vi "EKG.vi"() -> ()   [LabVIEW 2022 SP3]
uses:
  ViewData/-ReadEye/TypeDefs/TypeofMean.ctl
  <vilib>/Analysis/3filter.llb/Filter Passband Type.ctl
  <vilib>/Analysis/3filter.llb/Savitzky-Golay Filter (DBL).vi
  <vilib>/Analysis/baseanly.llb/Scale 1D.vi
  <vilib>/Utility/file.llb/Read Delimited Spreadsheet (string).vi
  <vilib>/picture/picture.llb/Draw True-Color Pixmap.vi
  <vilib>/Utility/file.llb/Write Delimited Spreadsheet (string).vi
  <vilib>/Analysis/NI_AAL_SigProc.lvlib
  <vilib>/Analysis/NI_AALBase.lvlib
panel:
  out "BPM file":string[][](array[string])
  out "clean lead 2 long":dbl[](graph)
  out "number of cycles":i32
  in  "Save?":bool
  out "clean lead 3":dbl[](graph)
  out "appended array":string[][](array[string])
  in  "Plot length":i32=3000
  in  "plot start":i32
  out "Input":dbl[](graph)
  out "Cycles":i32[](array[numeric])
  out "beats":i32
  in  "width":i32=10 min=3
  in  "Slide":dbl(slide)=0.5353535353535354 scale=0.0..1.0
  in  "slope correct?":bool
  in  "Process Path":path=path "\\\\vantage-n-wk\\H/Indus physiology recordings Fhf2 mouse"
  out "BPM":dbl
  in  "heartbeats":dbl=3.0
  out "Save Lead2":cluster{dbl[], "Y=(X-offset)/scale":dbl[]}(graph)
  out "clean Lead 3":cluster{dbl[], "Y=(X-offset)/scale":dbl[]}(graph)
  out "clean Lead 2":cluster{dbl[], "Y=(X-offset)/scale":dbl[]}(graph)
  out "Lead1":cluster{dbl[], "Y=(X-offset)/scale":dbl[]}(graph)
  in  "length":i32=6000
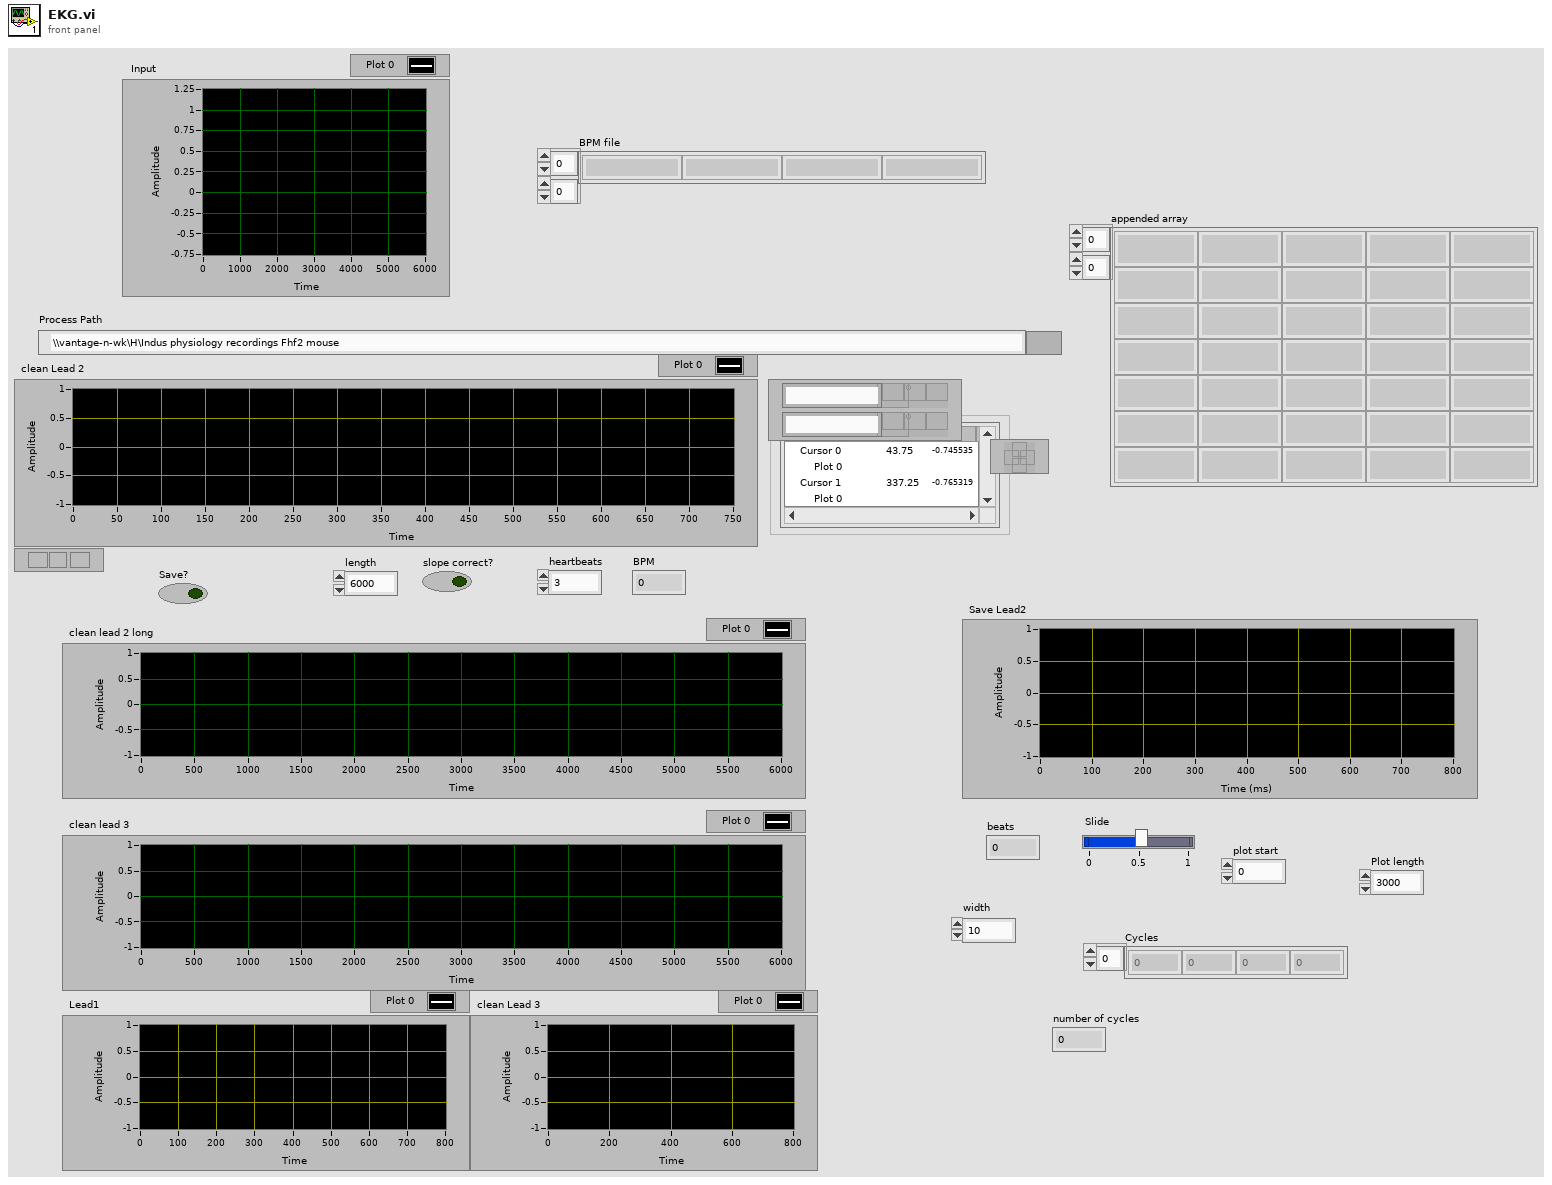
[diagram p1: front panel]
types:
  T1 = typedef "TypeofMean.ctl" = enum16{"Mean from lines", "Mean just lines", "Poly Mean", "No mean", "Filter"}
  T2 = typedef "NI_AALBase.lvlib/Filter Passband Type.ctl" = enum32{"Lowpass", "Highpass", "Bandpass", "Bandstop"}
  T3 = typedef "imagedata.ctl" = cluster{"image type":i32, "image depth":i32, "image":u8[], "mask":u8[], "colors":u32[], "Rectangle":cluster{"left":i16, "top":i16, "right":i16, "bottom":i16}}
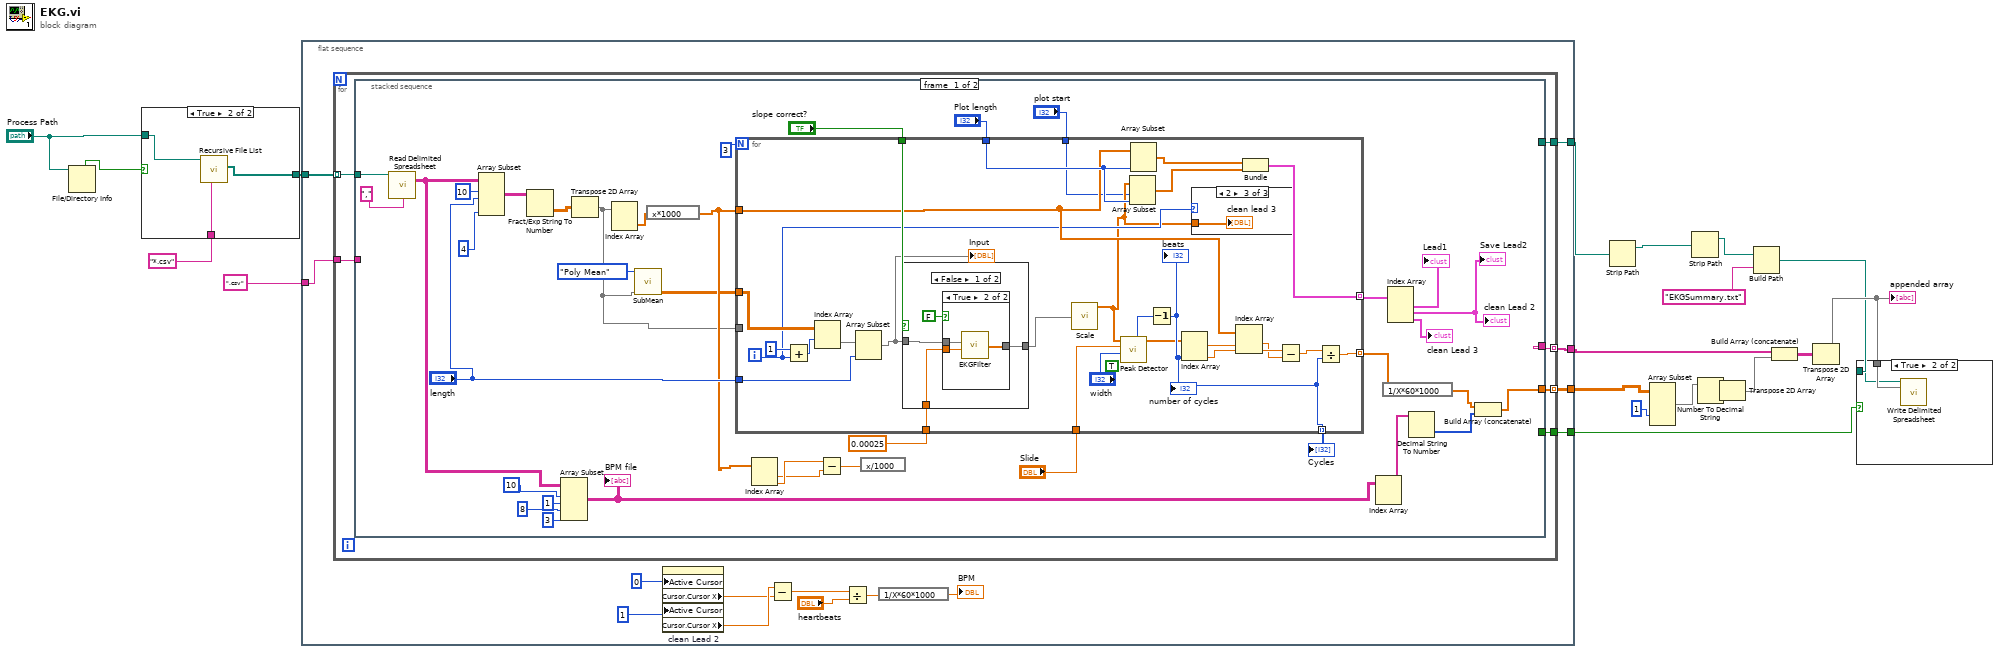
[diagram p0: block diagram]
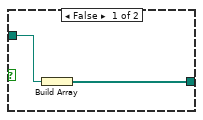
[diagram p3: hidden frame]
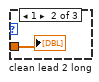
[diagram p5: hidden frame]
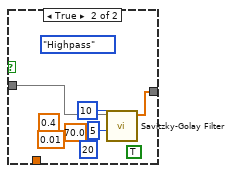
[diagram p7: hidden frame]
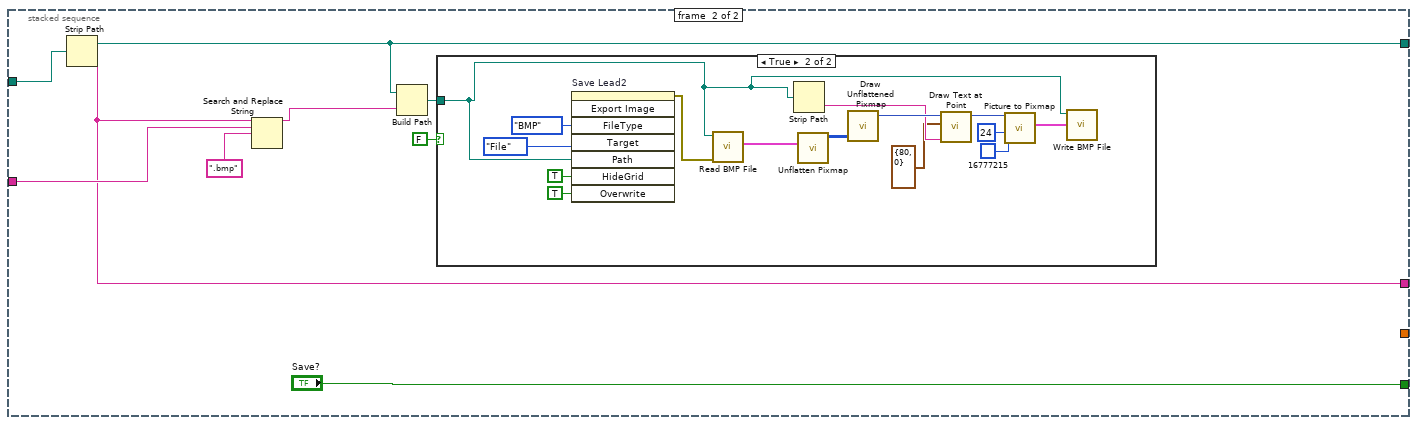
[diagram p8: hidden frame]
diagram:
  n1 = File/Directory Info(path="Process Path") -> (directory=w17:bool)  [unwired: 1 in, 6 out]
  n2 = case shown="True" w17 {
    tunnel: [w21 w24] -> w19
    tunnel: "Process Path" -> [w20 w23]
    tunnel: "*.csv" ("pattern") -> [_ w22]
    frame False {
      n3 = Build Array(w20) -> (w21:path[])
    }
    frame True {
      n4 = call <vilib>:"Recursive File List.vi"("pattern"=w22, "Folder Path"=w23) -> ("All Files in Dir"=w24:path[])  [unwired: 5 in, 4 out]
    }
  }
  n5 = flat-sequence {
    tunnel: w19 -> [w30]
    tunnel: [w26] -> w15
    tunnel: [w29] -> w14
    tunnel: [w28] -> w6
    tunnel: [w27] -> w2
    tunnel: ".csv" ("pattern") -> [w25]
    frame #0 {
      n6 = for {
        tunnel: w30 -> [w44] mode=indexing
        tunnel: [w43] -> w26 mode=indexing
        tunnel: w25 -> [w42]
        tunnel: [w41] -> w29 mode=indexing
        tunnel: [w40] -> w28
        tunnel: [w39] -> w27
        n7 = stacked-sequence {
          tunnel: w44 -> [w72 w132]
          tunnel: [w52 _] -> w43
          tunnel: w42 -> [_ w131]
          tunnel: [_ w127] -> w41
          tunnel: [_ w126] -> w40
          tunnel: [_ "Save?"] -> w39
          frame #0 {
            n8 = call-poly <vilib>:"Read Delimited Spreadsheet.vi"("file path (dialog if empty)"=w72, "delimiter (\\t)"="," ("delimiter (\\t)")) -> ("all rows"=w69:string[][])  [unwired: 8 in, 5 out]
            n9 = Array Subset(array=w69, index (row)=10 ("index"), length (row)="length", length (col)=4 ("length")) -> (w78:string[][])  [unwired: 1 in]
            n10 = Fract/Exp String To Number(string=w78) -> (number=w71:dbl[][])  [unwired: 3 in, 1 out]
            n11 = Array Subset(array=w69, index (row)=10, length (row)=1 ("length"), index (col)=8 ("disabled index (col)"), length (col)=3 ("length")) -> (w48:string[][])
            "BPM file" <- w48
            n12 = Transpose 2D Array(2D array=w71) -> (transposed array=w57:dbl[][])
            n13 = Index Array(array=w57) -> (element=w59:dbl[])  [unwired: 2 in]
            n14 = call "SubMean.vi"("Scan Data In"=w57, "Type of Mean"=TypeofMean."Poly Mean") -> ("Array"=w55:dbl[][])  [unwired: 4 in, 2 out]
            n15 = expression code="x*1000"(w59) -> (w58:dbl[])
            n16 = for {
              N: 3 -> [_]
              tunnel: w57 -> [_]
              tunnel: w58 -> [w88]
              tunnel: [w107] -> w76 mode=indexing
              tunnel: "length" -> [w105]
              tunnel: "slope correct?" -> [w104]
              tunnel: "Slide" -> [w103]
              tunnel: [w99] -> w66 mode=indexing
              tunnel: [w94] -> w65 mode=indexing
              tunnel: "plot start" -> [w83]
              tunnel: "Plot length" -> [w93]
              tunnel: 0.00025 -> [w82]
              tunnel: w55 -> [w86]
              i -> [w85]
              (unwired) TRUE ("initialize? (F)")
              n17 = Add(x=1, y=w85) -> (x+y=w108:i32)
              n18 = Index Array(array=w86, index (row)=w108) -> (element=w106:dbl[])  [unwired: 1 in]
              n19 = Array Subset(array=w106, length=w105) -> (w89:dbl[])  [unwired: 1 in]
              "Input" <- w89
              n20 = case shown="False" w104 {
                tunnel: [w114 w123] -> w87
                tunnel: w89 -> [w115 w122]
                tunnel: w82 -> [w113 _]
                frame False {
                  n21 = case shown="True" FALSE {
                    tunnel: w115 -> [w116 w119]
                    tunnel: [w116 w118] -> w114
                    tunnel: w113 -> [_ w117]
                    frame False {
                    }
                    frame True {
                      n22 = call "EKGFIlter.vi"("dt"=w117, "Input EKG"=w119) -> ("EKG Out"=w118:dbl[])  [unwired: 9 in]
                    }
                  }
                }
                frame True {
                  (unwired) 70.0 ("ripple(dB)")
                  (unwired) 20 ("order")
                  (unwired) 0.4 ("sampling freq: fs")
                  (unwired) TRUE ("init/cont (init:F)")
                  (unwired) 0.01 ("high cutoff freq: fh")
                  (unwired) Filter_Passband_Type."Highpass" ("filter type")
                  n23 = call-poly <vilib>:"Savitzky-Golay Filter.vi"("polynomial order"=5, "side points"=10, "X"=w122) -> ("Filtered X"=w123:dbl[])  [unwired: 7 in, 1 out]
                }
              }
              n24 = call-poly <vilib>:"Scale.vi"("X"=w87) -> ("Y=(X-offset)/scale"=w84:dbl[])  [unwired: 3 out]
              n25 = call <vilib>:"Peak Detector.vi"("width"="width", "threshold"=w103, "X"=w84) -> ("Locations"=w90:dbl[], "# found"=w101:i32)  [unwired: 4 in, 3 out]
              n26 = Array Subset(array=w84, index=w83, length=w93) -> (w91:dbl[])
              n27 = Array Subset(array=w88, length=w93) -> (w92:dbl[])  [unwired: 1 in]
              n28 = Decrement(x=w101) -> (x-1=w94:i32)
              "beats" <- w94
              n29 = Index Array(array=w90, index #2=w94) -> (element #1=w97:dbl, element #2=w98:dbl)  [unwired: 1 in]
              n30 = case shown="2" w85 {
                tunnel: w84 -> [_ w110 w111]
                frame 0, Default {
                }
                frame 1 {
                  "clean lead 2 long" <- w110
                }
                frame 2 {
                  "clean lead 3" <- w111
                }
              }
              n31 = Index Array(array=w88, index #1=w97, index #2=w98) -> (element #1=w95:dbl, element #2=w96:dbl)
              n32 = Bundle(w92, w91) -> (w107:cluster{dbl[], dbl[]})  [unwired: 1 in]
              n33 = Subtract(x=w96, y=w95) -> (x-y=w100:dbl)
              n34 = Divide(x=w100, y=w94) -> (x/y=w99:dbl)
            }
            "Cycles" <- w65
            n35 = Index Array(array=w58) -> (element #1=w60:dbl, element #2=w61:dbl)  [unwired: 2 in]
            n36 = Subtract(x=w61, y=w60) -> (x-y=w46:dbl)
            n37 = expression code="x/1000"(w46) -> ()  [unwired: 1 out]
            n38 = Index Array(array=w48) -> (element=w47:string[])  [unwired: 2 in]
            n39 = expression code="1/X*60*1000"(w66) -> (w54:dbl[])
            n40 = Index Array(array=w76) -> (element #1=→"Lead1":cluster{dbl[], dbl[]}, element #2=→"clean Lead 2" →"Save Lead2":cluster{dbl[], dbl[]}, element #3=→"clean Lead 3":cluster{dbl[], dbl[]})  [unwired: 3 in]
            n41 = Decimal String To Number(string=w47) -> (number=w53:i32[])  [unwired: 2 in, 1 out]
            n42 = Build Array (concatenate)(w54, w53) -> (w52:dbl[])
          }
          frame #1 {
            n43 = Strip Path(path=w132) -> (stripped path=w126:path, name=w127:string)
            n44 = Search and Replace String(input string=w127, search string=w131, replace string=".bmp" ("replace string (\"\")")) -> (result string=w129:string)  [unwired: 5 in, 3 out]
            n45 = Build Path(base path=w126, name or relative path=w129) -> (appended path=w128:path)
            n46 = case shown="True" FALSE {
              tunnel: w128 -> [_ w134]
              frame False {
              }
              frame True {
                n47 = invoke on="Save Lead2" class="XYGraph (strict)" method="Export Image"("FileType"=enum32{"BMP", "EPS", "EMF", "PICT"}."BMP" ("File Type"), "Target"=enum32{"File", "Clipboard"}."File", "Path"=w134, "HideGrid"=TRUE ("Hide Grid"), "Overwrite"=TRUE ("Always Overwrite")) -> (error out=w143:errorcluster)  [unwired: 3 in, 7 out]
                n48 = call <vilib>:"Read BMP File.vi"("error in (no error)"=w143, "path to BMP file"=w134) -> ("image data"=w141:T3)  [unwired: 7 in, 2 out]
                n49 = Strip Path(path=w134) -> (name=w139:string)  [unwired: 1 out]
                n50 = call <vilib>:"Unflatten Pixmap.vi"("image data"=w141) -> ("24-bit pixmap"=w142:u32[][])  [unwired: 4 in, 6 out]
                n51 = call-poly <vilib>:"Draw Unflattened Pixmap.vi"("data (RGB format)"=w142) -> ("new picture"=w140:picture)  [unwired: 8 in]
                n52 = call <vilib>:"Draw Text at Point.vi"("text"=w139, "origin"=cluster{"x":i16, "y":i16} {"x"=80, "y"=0}, "picture"=w140) -> ("new picture"=w138:picture)  [unwired: 7 in, 1 out]
                n53 = call <vilib>:"Picture to Pixmap.vi"("Background Color"=u32 16777215, "depth"=24, "picture"=w138) -> ("image data"=w135:T3)  [unwired: 7 in, 1 out]
                n54 = call <vilib>:"Write BMP File.vi"("image data"=w135, "path to BMP file"=w134) -> ()  [unwired: 8 in, 2 out]
              }
            }
          }
        }
      }
      n55 = property on="clean Lead 2" class="XYGraph (strict)"("Active Cursor"=u32 0, "Active Cursor"=u32 1) -> ("Cursor.Cursor X"=w35:dbl, "Cursor.Cursor X"=w36:dbl)  [unwired: 2 in, 2 out]
      n56 = Subtract(x=w36, y=w35) -> (x-y=w34:dbl)
      n57 = Divide(x=w34, y="heartbeats") -> (x/y=w32:dbl)
      n58 = expression code="1/X*60*1000"(w32) -> (→"BPM":dbl)
    }
  }
  n59 = Strip Path(path=w6) -> (stripped path=w7:path)  [unwired: 1 out]
  n60 = Array Subset(array=w15, index (col)=1 ("length")) -> (w13:dbl[][])  [unwired: 3 in]
  n61 = Strip Path(path=w7) -> (stripped path=w5:path)  [unwired: 1 out]
  n62 = Number To Decimal String(number=w13) -> (decimal integer string=w12:string[][])  [unwired: 1 in]
  n63 = Transpose 2D Array(2D array=w12) -> (transposed array=w10:string[][])
  n64 = Build Path(base path=w5, name or relative path="EKGSummary.txt") -> (appended path=w3:path)
  n65 = Build Array (concatenate)(w14, w10) -> (w11:string[][])
  n66 = Transpose 2D Array(2D array=w11) -> (transposed array=w8:string[][])
  "appended array" <- w8
  n67 = case shown="True" w2 {
    tunnel: w8 -> [_ w149]
    tunnel: w3 -> [_ w148]
    frame False {
    }
    frame True {
      n68 = call-poly <vilib>:"Write Delimited Spreadsheet.vi"("file path (dialog if empty)"=w148, "2D data"=w149) -> ()  [unwired: 12 in, 2 out]
    }
  }
